vi "Parse EscapedVariable.vi"(8 "Error In":errorcluster) -> (0 "Error Out":errorcluster)   [LabVIEW 2018, in "Tests.lvlib" / "Parser.lvlib"]
uses:
  Parser.lvlib
  src/Toolkit/Tokens/EscapedVariable/EscapedVariable.lvclass
  src/Toolkit/Tokens/Keyable/API/Keyable.lvclass/Keyable.ctl
  src/Toolkit/Tokens/Keyable/API/Read Key.vi
  src/Toolkit/Readers/String/String.lvclass
  D:/Users/cfield/Code/Field R&D Services/Mustache/trunk/src/Toolkit/Readers/Abstract/Abstract.lvclass
  <vilib>/Utility/LVClass/Get LV Class Name.vi
  src/Toolkit/Tokens/Keyable/API/Keyable.lvclass
  <vilib>/addons/_JKI Toolkits/Caraya/classes/Test/Test.lvclass
  src/Toolkit/Parser/Parser.lvclass
  <vilib>/addons/_JKI Toolkits/Caraya/classes/Assert/Assert.lvclass
  Tests.lvlib
  src/Toolkit/Tokens/Abstract/Abstract.lvclass
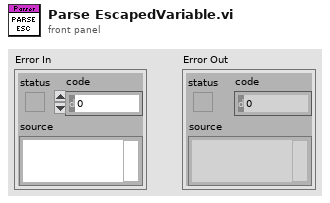
[diagram p1: front panel]
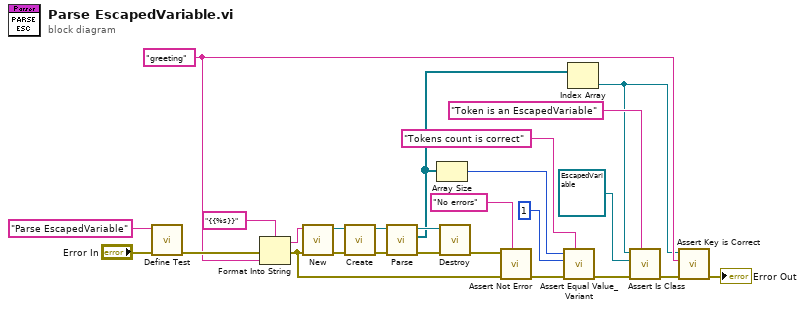
[diagram p0: block diagram]
diagram:
  w2 = "greeting"
  n1 = call <vilib>:"Define Test.vi"("error in (no error)"="Error In", "Label (VI Title)"="Parse EscapedVariable") -> ("error out"=w17:errorcluster)  [unwired: 9 in]
  n2 = Format Into String(format string="{{%s}}", error in=w17, w2) -> (resulting string=w5:string, error out=w7:errorcluster)  [unwired: 1 in]
  n3 = call "New.vi"("Error In"=w7, "String"=w5) -> ("Error Out"=w23:errorcluster, "String"=w24:refnum<class "String.lvclass">)  [unwired: 8 in]
  n4 = call "Create.vi"("Error In"=w23, "Reader"=w24) -> ("Error Out"=w22:errorcluster, "Parser"=w21:refnum<class "Parser.lvclass">)  [unwired: 8 in]
  n5 = call "Parse.vi"("Error In"=w22, "Parser In"=w21) -> ("Error Out"=w19:errorcluster, "Tokens"=w11:refnum<class "Abstract.lvclass">[], "Parser Out"=w20:refnum<class "Parser.lvclass">)  [unwired: 7 in]
  n6 = Array Size(array=w11) -> (size(s)=w13:i32)
  n7 = call "Destroy.vi"("Error In"=w19, "Parser"=w20) -> ("Error Out"=w18:errorcluster)  [unwired: 9 in]
  n8 = call <vilib>:"Assert Not Error.vi"("Label"="No errors", "error in (no error)"=w7, "Not Error?"=w18) -> ("error out"=w15:errorcluster)  [unwired: 8 in]
  n9 = call <vilib>:"Assert Equal Value_Variant.vi"("Label"="Tokens count is correct", "error in (no error)"=w15, "Y"=1 ("size(s)"), "X"=w13) -> ("error out"=w10:errorcluster)  [unwired: 7 in]
  n10 = Index Array(array=w11) -> (element=w1:refnum<class "Abstract.lvclass">)  [unwired: 1 in]
  n11 = call "Assert Is Class.vi"("Label"="Token is an EscapedVariable", "Error In"=w10, "Expected"=refnum<class "EscapedVariable.lvclass"> refnum ("Mustache.lvlib:Tokens.lvlib:EscapedVariable.lvclass"), "Actual"=w1) -> ("Error Out"=w8:errorcluster)  [unwired: 7 in]
  n12 = call "Assert Key is Correct.vi"("Error In"=w8, "Expected"=w2, "Token"=w1) -> ("Error Out"=→"Error Out":errorcluster)  [unwired: 8 in]
